vi "Select Scope.vi"(8 "Error In":errorcluster, 10 "Strings[]":string[](array[string]), 11 "App In":refnum<vi>) -> (0 "Error Out":errorcluster, 2 "Selection":u16, 3 "App Out":refnum<vi>)   [LabVIEW 2017, in "Graveyard.lvlib"]
uses:
  Graveyard.lvlib
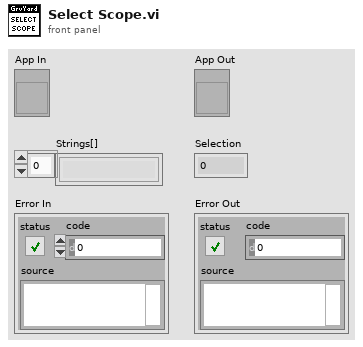
[diagram p1: front panel]
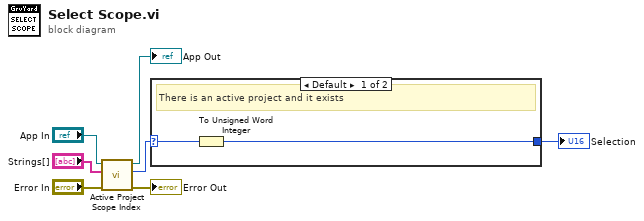
[diagram p0: block diagram]
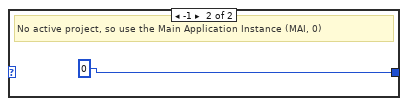
[diagram p2: hidden frame]
diagram:
  n1 = call "Active Project Scope Index.vi"("Error In"="Error In", "Strings[]"="Strings[]", "App In"="App In") -> ("Error Out"=→"Error Out":errorcluster, "Index"=w4:i32, "App Out"=→"App Out":refnum<vi>)  [unwired: 6 in]
  n2 = case shown="Default" w4 {
    selector: w4 -> [w8 _]
    tunnel: [w9 u16 0] -> w3
    frame Default {
      # "There is an active project and it exists"
      n3 = To Unsigned Word Integer(number=w8) -> (unsigned 16bit integer=w9:u16)
    }
    frame -1 {
      # "No active project, so use the Main Application Instance (MAI, 0)"
    }
  }
  "Selection" <- w3
